vi "Load DAC Configuration.vi"(8 "error in":errorcluster, 10 "Config File refnum in":T1, 11 "DAC FTCU in":refnum<class "DAC FTCU.lvclass">) -> (0 "error out":errorcluster, 2 "Config File refnum out":T1, 3 "DAC FTCU out":refnum<class "DAC FTCU.lvclass">)   [LabVIEW 2019, in "DAC.lvlib" / "DAC FTCU.lvclass"]
uses:
  DAC FTCU.lvclass
  <vilib>/Utility/config.llb/Config Data RefNum.ctl
  DAC.lvclass
  <vilib>/Utility/config.llb/NI_LVConfig.lvlib
  <vilib>/Utility/config.llb/Read Key (String).vi
  C:/Users/krio/Documents/LV_Projects/test-stand/App/DAC/DAC.lvclass
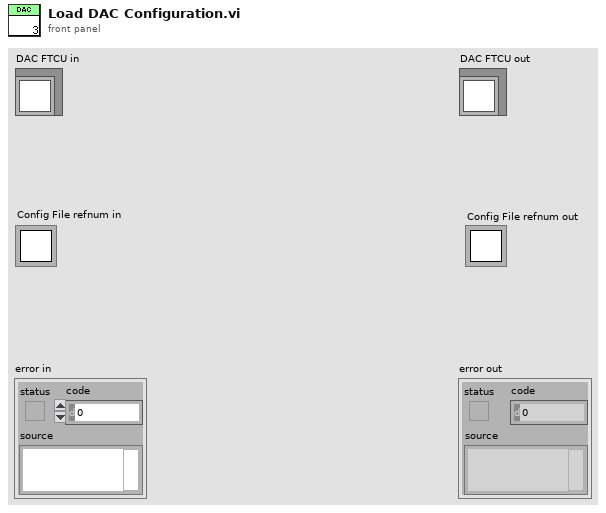
[diagram p1: front panel]
types:
  T1 = typedef "NI_LVConfig.lvlib/Config Data RefNum.ctl" = refnum<k1>
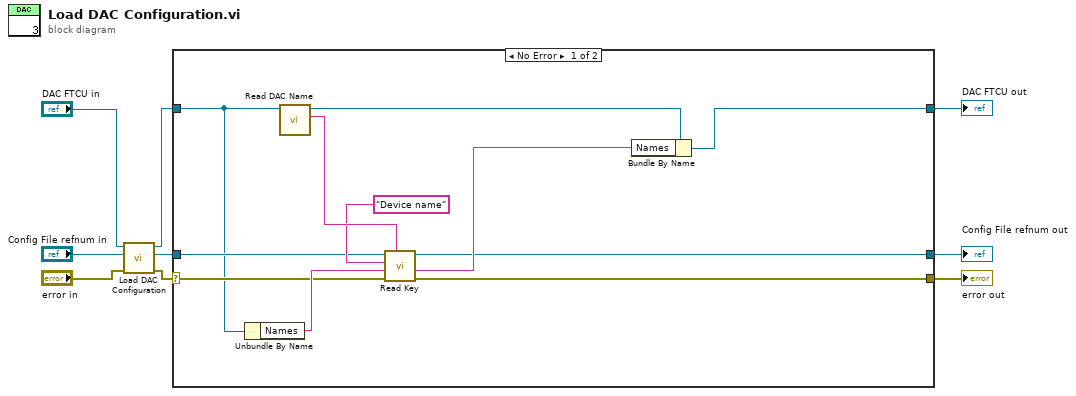
[diagram p0: block diagram]
diagram:
  n1 = call-parent "Load DAC Configuration.vi"("error in"="error in", "Config File refnum in"="Config File refnum in", "DAC in"="DAC FTCU in") -> ("error out"=w4:errorcluster, "Config File refnum out"=w5:T1, "DAC out"=w6:refnum<class "DAC FTCU.lvclass">)  [unwired: 6 in]
  n2 = case shown="No Error" w4 {
    selector: w4 -> [w14 w23]
    tunnel: [w10 w23] -> w1
    tunnel: [w12 w22] -> w3
    tunnel: w6 -> [w13 w22]
    tunnel: w5 -> [w15 w21]
    tunnel: [w11 w21] -> w2
    frame No Error {
      n3 = Unbundle By Name(w13) -> ("Names"=w18:string)
      n4 = call "Read DAC Name.vi"("DAC in"=w13) -> ("DAC Name"=w20:string, "DAC out"=w17:refnum<class "DAC FTCU.lvclass">)  [unwired: 8 in, 1 out]
      n5 = call-poly <vilib>:"Read Key.vi"("section"=w20, "error in (no error)"=w14, "default value"=w18, "key"="Device name", "refnum"=w15) -> ("error out"=w10:errorcluster, "value"=w16:string, "refnum out"=w11:T1)  [unwired: 3 in, 1 out]
      n6 = Bundle By Name(cluster=w17, "Names"=w16) -> (w12:refnum<class "DAC FTCU.lvclass">)
    }
    frame Error {
    }
  }
  "error out" <- w1
  "DAC FTCU out" <- w3
  "Config File refnum out" <- w2
